vi "inject-spur.vi"(6 "Harmonics in":T2(array[cluster]), 9 "inject-harmonic":bool, 10 "index (row)":i32, 11 "Harmonics 3":T1(array[cluster])) -> (3 "Harmonics out":T1(array[cluster]))   [LabVIEW 2024]
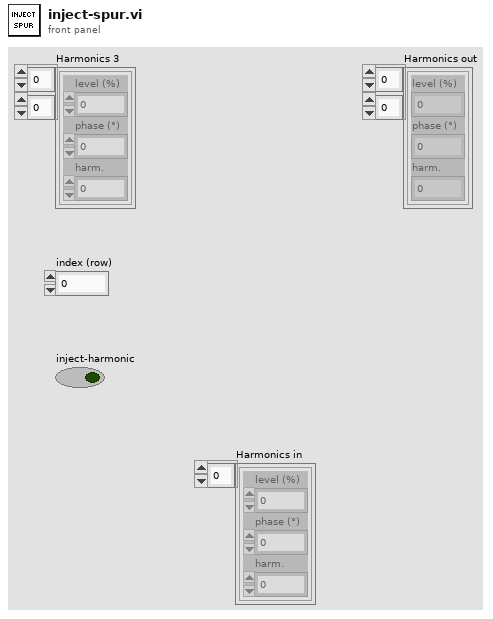
[diagram p1: front panel]
types:
  T1 = cluster{"level (%)":dbl, "phase (°)":dbl, "harm.":dbl}[][]
  T2 = cluster{"level (%)":dbl, "phase (°)":dbl, "harm.":dbl}[]
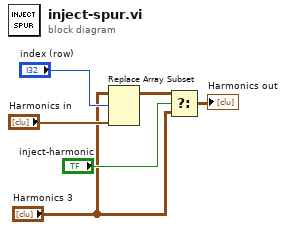
[diagram p0: block diagram]
diagram:
  n1 = Replace Array Subset(array="Harmonics 3", new element="Harmonics in", index (row)="index (row)") -> (w1:T1)  [unwired: 1 in]
  n2 = Select(t=w1, s="inject-harmonic", f="Harmonics 3") -> (s? t:f=→"Harmonics out":T1)
